vi "Test_Averaging.vi"() -> ()   [LabVIEW 2022 SP3]
panel:
  in  "Slide Window L":i32=3 min=3 max=100 step=2
  in  "Ampl. Shot Noise, 0...1":dbl=1.2000000000000006 min=0.0 max=1.25 step=0.05
  in  "Amplitude Signal":dbl=1.0 min=1.0 max=10.0 step=1.0
  in  "Stop":bool
  in  "Generate Sine":bool
  out "Signal":dbl[][](graph)
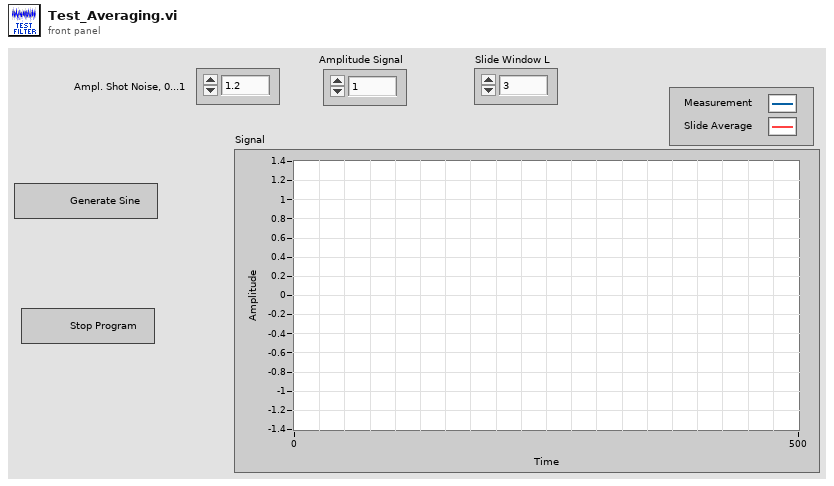
[diagram p1: front panel]
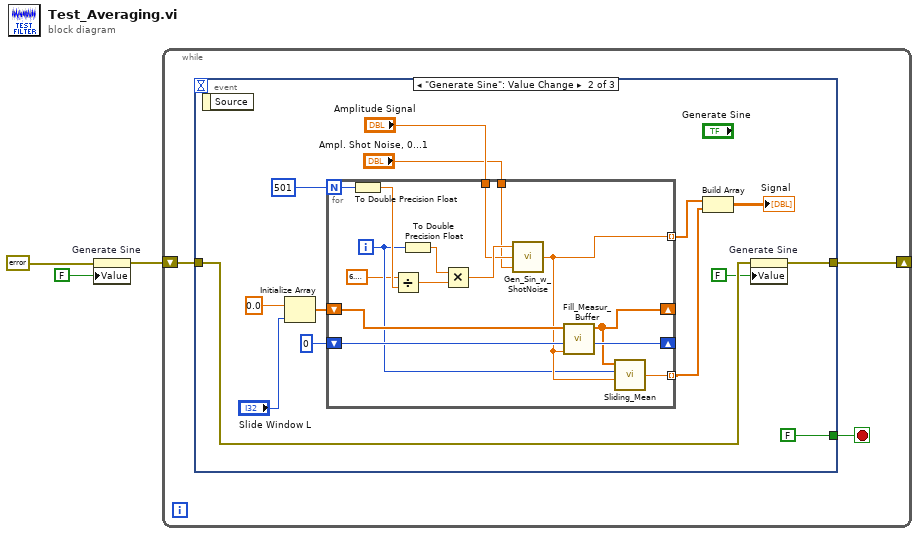
[diagram p0: block diagram]
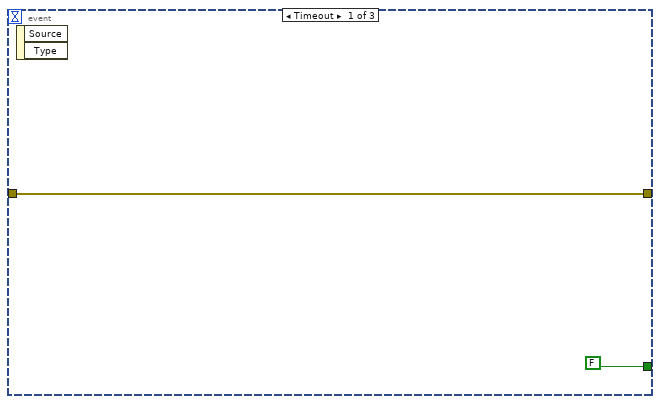
[diagram p2: hidden frame]
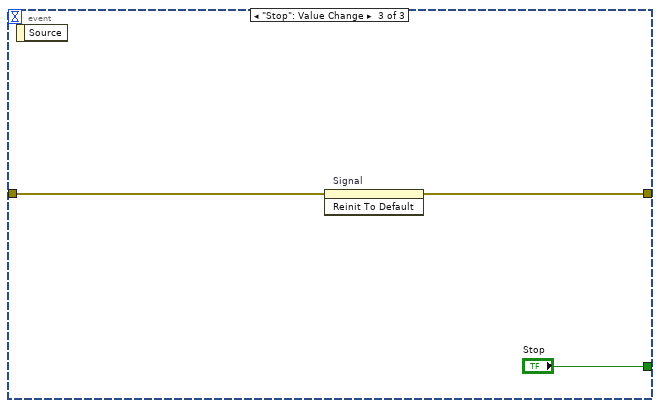
[diagram p3: hidden frame]
diagram:
  n1 = property on="Generate Sine" class="Bool (strict)"(error in=errorcluster {"status"=FALSE, "code"=0, "source"=""} ("error in (no error)"), "Value"=FALSE ("Generate Sine")) -> (error out=w2:errorcluster)  [unwired: 1 in, 1 out]
  n2 = while {
    shift-right: [w4] -> _
    shift-left: w2 -> [w5]
    stop <- w6 stop-if-true
    n3 = event shown="[1] \"Generate Sine\": Value Change" {
      selector: _ -> [_ _ _]
      dyn-events: _ -> [_ _ _]
      timeout: _ -> [_ _ _]
      tunnel: [FALSE ("Stop") FALSE ("Stop") "Stop"] -> w6
      tunnel: w5 -> [w7 w19 w39]
      tunnel: [w7 w20 w38] -> w4
      event Timeout {
        n4 = event-data() -> ()  [unwired: 1 in, 2 out]
      }
      event "Generate Sine": Value Change {
        n5 = event-data() -> ()  [unwired: 1 in, 1 out]
        n6 = Initialize Array(0.0 ("element"), "Slide Window L") -> (w11:dbl[])
        n7 = for {
          N: 501 -> [w37]
          tunnel: [w27] -> w14 mode=indexing
          tunnel: "Amplitude Signal" -> [w32]
          tunnel: "Ampl. Shot Noise, 0...1" -> [w31]
          shift-right: [w29] -> _
          shift-left: 0 -> [w30]
          shift-right: [w26] -> _
          shift-left: w11 -> [w28]
          tunnel: [w25] -> w13 mode=indexing
          i -> [w24]
          n8 = To Double Precision Float(number=w37) -> (double precision float=w36:dbl)
          n9 = Divide(x=6.283185307179586, y=w36) -> (x/y=w34:dbl)
          n10 = To Double Precision Float(number=w24) -> (double precision float=w35:dbl)
          n11 = Multiply(x=w35, y=w34) -> (x*y=w33:dbl)
          n12 = call "Gen_Sin_w_ShotNoise.vi"("[IN] Ampl. Shot Noise, 0...1"=w31, "[IN] Amplitude"=w32, "[IN] X value"=w33) -> ("[OUT] Value"=w27:dbl)  [unwired: 1 in]
          n13 = call "Fill_Measur_Buffer.vi"("[IN] Current Measure"=w27, "[IN] Current Index"=w30, "[IN] Buffer"=w28) -> ("[OUT] Current Index"=w29:i32, "[OUT] Buffer"=w26:dbl[])  [unwired: 3 in]
          n14 = call "Sliding_Mean.vi"("[IN] Buffer"=w26, "[IN] Iteration / # Measurment"=w24, "[IN] Current Measure"=w27) -> ("[OUT] Sliding Average"=w25:dbl)  [unwired: 2 in]
        }
        n15 = Build Array(w14, w13) -> (→"Signal":dbl[][])
        n16 = property on="Generate Sine" class="Bool (strict)"(error in=w19, "Value"=FALSE ("Generate Sine")) -> (error out=w20:errorcluster)  [unwired: 1 in, 1 out]
      }
      event "Stop": Value Change {
        n17 = event-data() -> ()  [unwired: 1 in, 1 out]
        n18 = invoke on="Signal" class="WFGraph (strict)" method="Reinit To Default"(error in=w39) -> (error out=w38:errorcluster)  [unwired: 2 in, 2 out]
      }
    }
  }
